vi "start.vi"(8 "error in (no error)":errorcluster, 11 "Hamamatsu_C9100-13 in":refnum<class "Hamamatsu_C9100-13.lvclass">) -> (0 "error out":errorcluster, 3 "Hamamatsu_C9100-13 out":refnum<class "Hamamatsu_C9100-13.lvclass">)   [LabVIEW 2013, in "Hamamatsu_C9100-13.lvclass"]
uses:
  Hamamatsu_C9100-13.lvclass
  Hamamatsu_C9100-13.lvclass/Hamamatsu_C9100-13.ctl
  Experiment/Globals.vi
panel:
  out "Acquiring?":bool
  out "Trigger mode after IMAQ start":string
  out "Last Valid Buffer Number":i32
  out "IMAQ Session Out":refnum<k11>
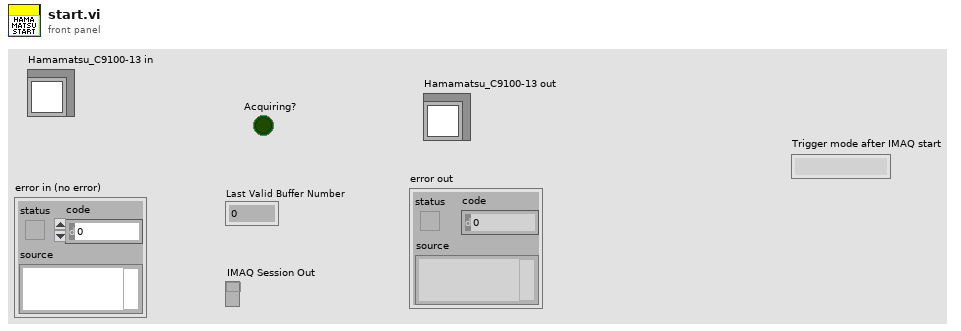
[diagram p1: front panel]
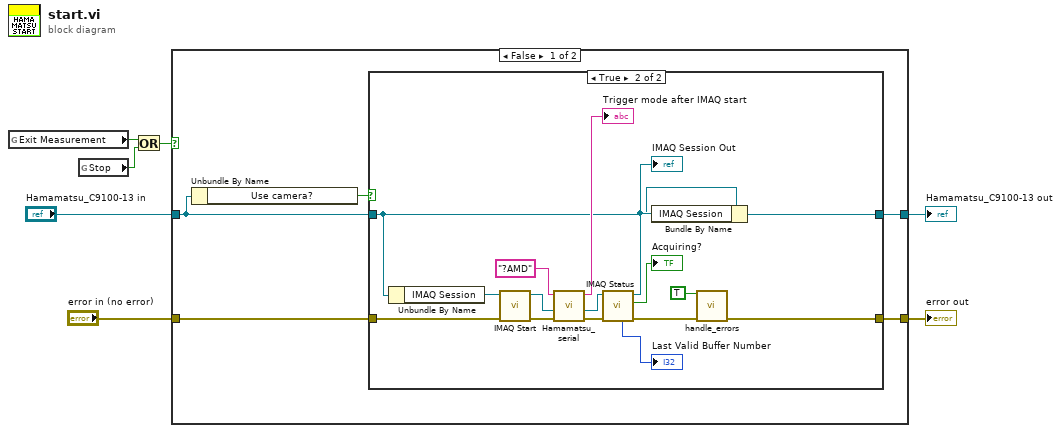
[diagram p0: block diagram]
diagram:
  n1 = global read "Globals.vi" "Exit Measurement"() -> (w2:bool)
  n2 = global read "Globals.vi" "Stop"() -> (w3:bool)
  n3 = Or(x=w2, y=w3) -> (x .or. y?=w1:bool)
  n4 = case shown="False" w1 {
    tunnel: [w12 w31] -> w7
    tunnel: [w11 w32] -> w6
    tunnel: "Hamamatsu_C9100-13 in" -> [w9 w32]
    tunnel: "error in (no error)" -> [w10 w31]
    frame False {
      n5 = Unbundle By Name(w9) -> ("Use camera?"=w8:bool)
      n6 = case shown="True" w8 {
        tunnel: [w13 w17] -> w12
        tunnel: [w14 w19] -> w11
        tunnel: w9 -> [w14 w16]
        tunnel: w10 -> [w13 w18]
        frame False {
        }
        frame True {
          n7 = Unbundle By Name(w16) -> ("IMAQ Session"=w15:refnum<k11>)
          n8 = call <vilib>:"IMAQ Start.vi"("error in (no error)"=w18, "IMAQ Session In"=w15) -> ("error out"=w21:errorcluster, "IMAQ Session Out"=w20:refnum<k11>)  [unwired: 8 in]
          n9 = call "Hamamatsu_serial.vi"("error in"=w21, "IMAQ Session In"=w20, "Command to send"="?AMD") -> ("error out"=w27:errorcluster, "IMAQ Session Out"=w26:refnum<k11>, "Response from Camera"=→"Trigger mode after IMAQ start":string)  [unwired: 6 in]
          n10 = call <vilib>:"IMAQ Status.vi"("error in (no error)"=w27, "IMAQ Session In"=w26) -> ("error out"=w22:errorcluster, "Acquiring?"=→"Acquiring?":bool, "IMAQ Session Out"=w25:refnum<k11>, "Last Valid Buffer Number"=→"Last Valid Buffer Number":i32)  [unwired: 5 in, 1 out]
          "IMAQ Session Out" <- w25
          n11 = Bundle By Name(cluster=w16, "IMAQ Session"=w25) -> (w19:refnum<class "Hamamatsu_C9100-13.lvclass">)
          n12 = call "handle_errors.vi"("Exit Operation"=TRUE, "error in (no error)"=w22) -> ("error out"=w17:errorcluster)  [unwired: 13 in]
        }
      }
    }
    frame True {
    }
  }
  "error out" <- w7
  "Hamamatsu_C9100-13 out" <- w6
